vi "PCert-Application-Directories.vi"(8 "error in":errorcluster) -> (0 "error out":errorcluster, 2 "Provider Root":path, 3 "Deploy Root":path)   [LabVIEW 2013]
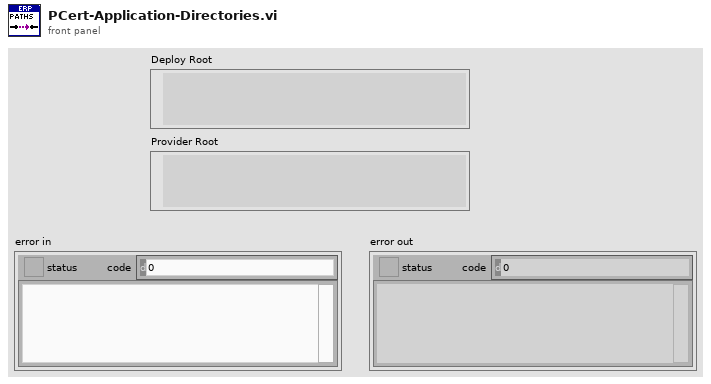
[diagram p1: front panel]
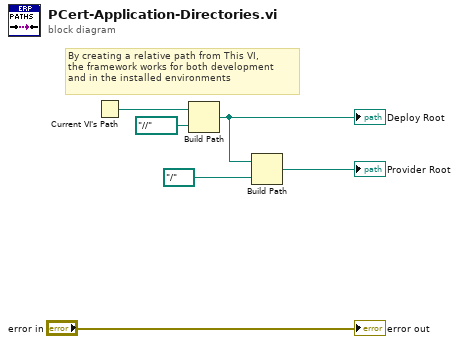
[diagram p0: block diagram]
diagram:
  # "By creating a relative path from This VI,\nthe framework works for both development\nand in the installed environments"
  n1 = Current VI's Path() -> (path=w1:path)
  n2 = Build Path(base path=w1, name or relative path=path "../../..") -> (appended path=w4:path)
  "Deploy Root" <- w4
  n3 = Build Path(base path=w4, name or relative path=path "../..") -> (appended path=→"Provider Root":path)
  "error out" <- "error in"
